vi "Group Traces.vi"(7 "Mean":bool, 8 "Plot Selection 2":T1(array[cluster]), 9 "Channels / Subject":T3(array[cluster]) {"Offset" format="%.2f"}, 10 "Data Input":T2(array[cluster]) {"Data Channels" format="%.2f"}) -> (0 "STD":dbl[][](array[numeric]) format="%.2f", 1 "Mean":dbl[][](array[numeric]) format="%.2f", 3 "Output":dbl[][](array[numeric]) format="%.2f")   [LabVIEW 2013]
uses:
  comm/stats/stats.lvlib
  comm/nan operations/nan operations.lvlib
panel:
  # "Copyright Americo A. Migliaccio (c) 2002 All Rights Reserved by Author"
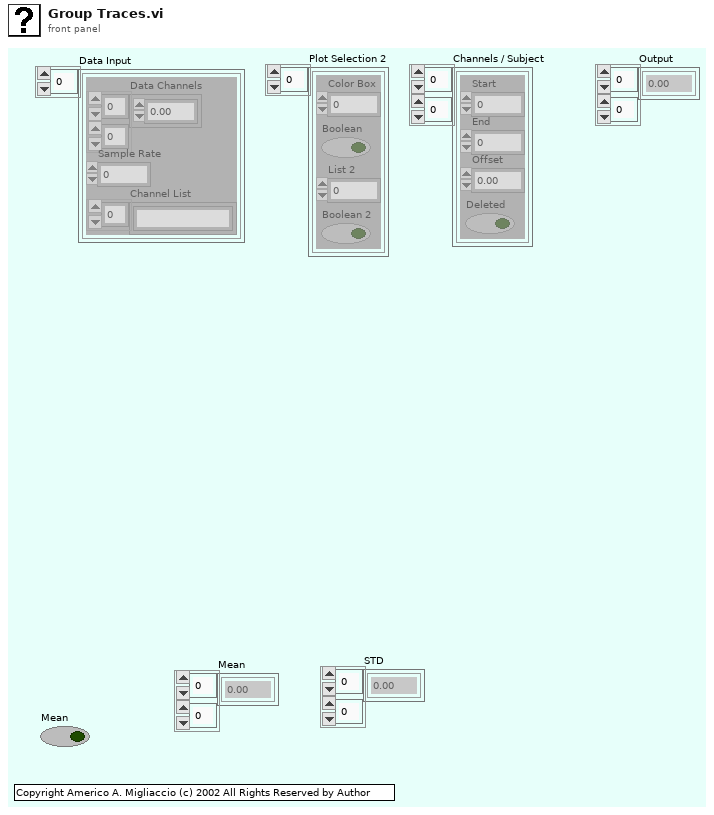
[diagram p1: front panel]
types:
  T1 = cluster{"Color Box":u32, "Boolean":bool, "List 2":u16, "Boolean 2":bool}[]
  T2 = cluster{"Data Channels":dbl[][], "Sample Rate":i32, "Channel List":string[]}[]
  T3 = cluster{"Start":i32, "End":i32, "Offset":dbl, "Deleted":bool}[][]
  T4 = cluster{"Start":i32, "End":i32, "Offset":dbl, "Deleted":bool}
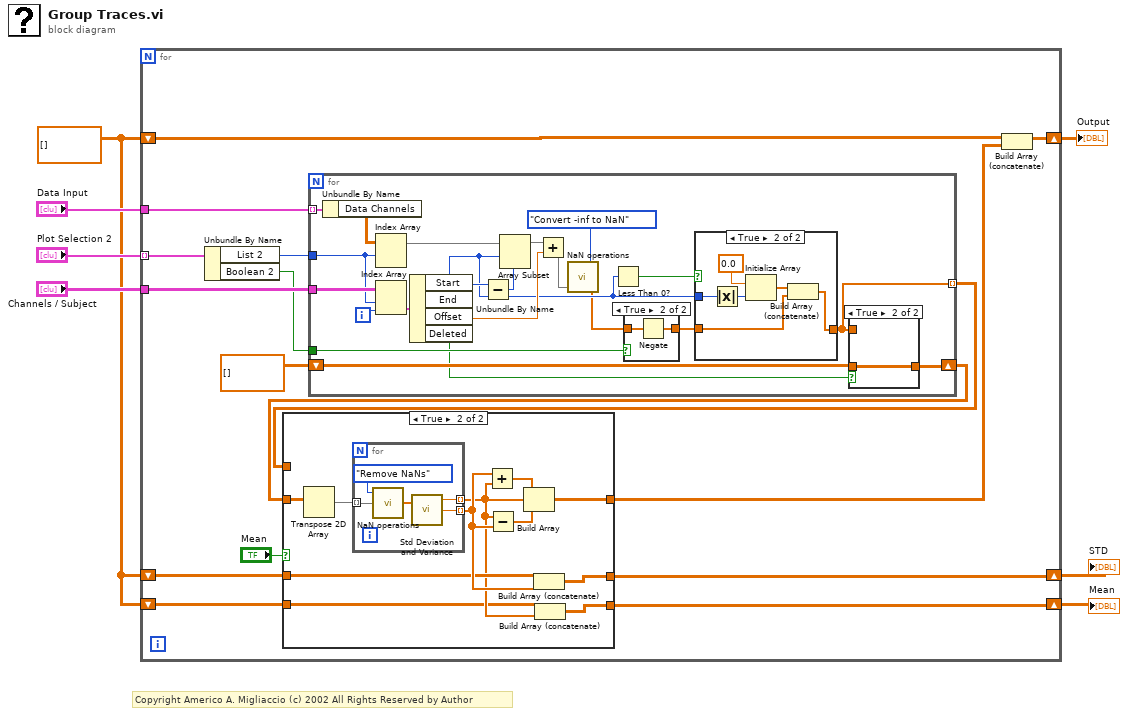
[diagram p0: block diagram]
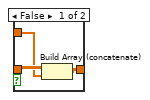
[diagram p3: hidden frame]
diagram:
  w3 = dbl[][] []
  # "Copyright Americo A. Migliaccio (c) 2002 All Rights Reserved by Author"
  n1 = for {
    tunnel: "Plot Selection 2" -> [w23] mode=indexing
    tunnel: "Channels / Subject" -> [w20]
    tunnel: "Data Input" -> [w22]
    shift-right: [w19] -> w5
    shift-left: w3 -> [w18]
    shift-right: [w9] -> w2
    shift-left: w3 -> [w11]
    shift-right: [w8] -> w1
    shift-left: w3 -> [w10]
    n2 = Unbundle By Name(w23) -> ("List 2"=w21:u16, "Boolean 2"=w17:bool)
    n3 = for {
      tunnel: w22 -> [w64] mode=indexing
      tunnel: w21 -> [w54]
      tunnel: w20 -> [w62]
      tunnel: w17 -> [w52]
      shift-right: [w50] -> w13
      shift-left: dbl[][] [] -> [w51]
      tunnel: [w46] -> w12 mode=indexing
      i -> [w55]
      n4 = Unbundle By Name(w64) -> ("Data Channels"=w63:dbl[][])
      n5 = Index Array(array=w63, index (row)=w54) -> (element=w60:dbl[])  [unwired: 1 in]
      n6 = Index Array(array=w62, index (row)=w54, index (col)=w55) -> (element=w61:T4)
      n7 = Unbundle By Name(w61) -> ("Start"=w53:i32, "End"=w59:i32, "Offset"=w57:dbl, "Deleted"=w47:bool)
      n8 = Subtract(x=w59, y=w53) -> (x-y=w58:i32)
      n9 = Array Subset(array=w60, index=w53, length=w58) -> (w56:dbl[])
      n10 = Add(x=w56, y=w57) -> (x+y=w44:dbl[])
      n11 = call "NaN operations.vi"("Data(in)"=w44, "Operation"=enum16{"Remove NaNs", "Convert -inf to NaN"}."Convert -inf to NaN") -> ("Data(out)"=w45:dbl[])  [unwired: 3 in]
      n12 = Less Than 0?(x=w53) -> (x < 0?=w49:bool)
      n13 = case shown="True" w52 {
        tunnel: w45 -> [w69 w71]
        tunnel: [w69 w70] -> w48
        frame False {
        }
        frame True {
          n14 = Negate(x=w71) -> (-x=w70:dbl[])
        }
      }
      n15 = case shown="True" w49 {
        tunnel: w53 -> [_ w78]
        tunnel: w48 -> [w72 w74]
        tunnel: [w72 w73] -> w46
        frame False {
        }
        frame True {
          n16 = Absolute Value(x=w78) -> (abs(x)=w77:i32)
          n17 = Initialize Array(0.0 ("Element Data"), w77) -> (w75:dbl[])
          n18 = Build Array (concatenate)(w75, w74) -> (w73:dbl[])
        }
      }
      n19 = case shown="True" w47 {
        tunnel: w51 -> [w66 w68]
        tunnel: [w67 w68] -> w50
        tunnel: w46 -> [w65 _]
        frame False {
          n20 = Build Array (concatenate)(w66, w65) -> (w67:dbl[][])
        }
        frame True {
        }
      }
    }
    n21 = case shown="True" "Mean" {
      tunnel: w13 -> [_ w34]
      tunnel: [w26 w33] -> w15
      tunnel: w12 -> [w26 _]
      tunnel: w11 -> [w25 w31]
      tunnel: w10 -> [w24 w29]
      tunnel: [w25 w28] -> w9
      tunnel: [w24 w27] -> w8
      frame False {
      }
      frame True {
        n22 = Transpose 2D Array(2D array=w34) -> (transposed array=w35:dbl[][])
        n23 = for {
          tunnel: w35 -> [w39] mode=indexing
          tunnel: [w42] -> w30 mode=indexing
          tunnel: [w41] -> w32 mode=indexing
          n24 = call "NaN operations.vi"("Data(in)"=w39, "Operation"=enum16{"Remove NaNs", "Convert -inf to NaN"}."Remove NaNs") -> ("Data(out)"=w40:dbl[])  [unwired: 3 in]
          n25 = call "Std Deviation and Variance.vi"("X"=w40) -> ("mean"=w42:dbl, "standard deviation"=w41:dbl)  [unwired: 1 in, 1 out]
        }
        n26 = Add(x=w32, y=w30) -> (x+y=w37:dbl[])
        n27 = Subtract(x=w30, y=w32) -> (x-y=w36:dbl[])
        n28 = Build Array(w37, w30, w36) -> (w33:dbl[][])
        n29 = Build Array (concatenate)(w31, w32) -> (w28:dbl[][])
        n30 = Build Array (concatenate)(w29, w30) -> (w27:dbl[][])
      }
    }
    n31 = Build Array (concatenate)(w18, w15) -> (w19:dbl[][])
  }
  "Output" <- w5
  "Mean" <- w1
  "STD" <- w2
